vi "Mix List.vi"(0 "List in":string[](array[string]), 1 "List Order":map{i32, string}(c390), 2 "#Mix":i32=1) -> (3 "List out":string[](array[string]))   [LabVIEW 2020, in "AoC 2022.lvlib"]
uses:
  AoC 2022.lvlib
  fe89e87c-1a3d-4cd6-ae88-14682854c04f.vi
  1fd5187e-c1bf-43b5-9c42-e30538a947da.vi
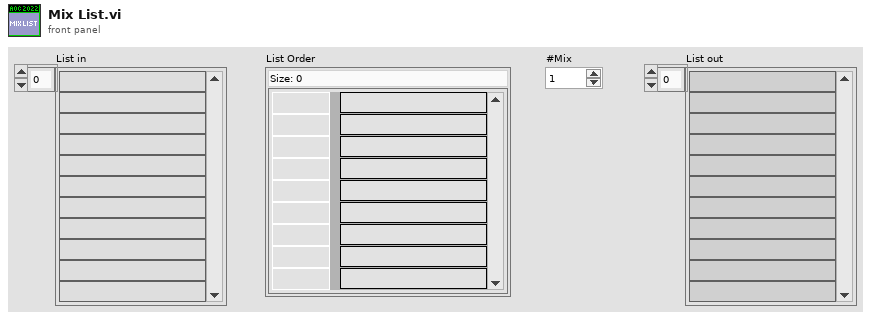
[diagram p1: front panel]
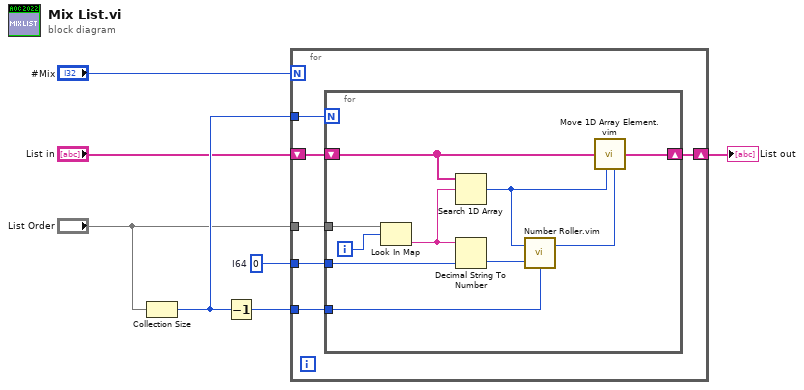
[diagram p0: block diagram]
diagram:
  w7 = i64 0  # I64
  n1 = Collection Size(1:"List Order") -> (0:w6:i32)
  n2 = Decrement(x=w6) -> (x-1=w5:i32)
  n3 = for {
    N: "#Mix" -> [_]
    tunnel: w7 -> [w13]
    tunnel: w6 -> [w12]
    tunnel: w5 -> [w11]
    tunnel: "List Order" -> [w9]
    shift-right: [w10] -> w4
    shift-left: "List in" -> [w8]
    n4 = for {
      N: w12 -> [_]
      shift-right: [w16] -> w10
      shift-left: w8 -> [w23]
      tunnel: w9 -> [w21]
      tunnel: w11 -> [w18]
      tunnel: w13 -> [w14]
      i -> [w20]
      n5 = Look In Map(map=w21, key=w20) -> (value=w19:string)  [unwired: 1 in, 1 out]
      n6 = Search 1D Array(1D array=w23, element=w19) -> (index of element=w22:i32)  [unwired: 1 in]
      n7 = Decimal String To Number(string=w19, default (0L)=w14) -> (number=w17:i64)  [unwired: 1 in, 1 out]
      n8 = call "Number Roller.vim"("Current Value"=w22, "Max Range"=w18, "Movement"=w17) -> ("Next Value"=w15:i64)  [unwired: 1 out]
      n9 = call "Move 1D Array Element.vim"("Array in"=w23, "From Index"=w22, "To Index"=w15) -> ("Array out"=w16:string[])
    }
  }
  "List out" <- w4
